vi "Controller Request PS Setpoints.vi"(8 "error in":errorcluster, 11 "Return All Setpoints":bool) -> (0 "error out":errorcluster)   [LabVIEW 2011, in "Controller VIs.lvlib"]
uses:
  Controller VIs.lvlib
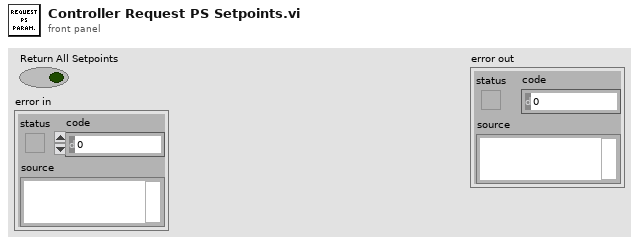
[diagram p1: front panel]
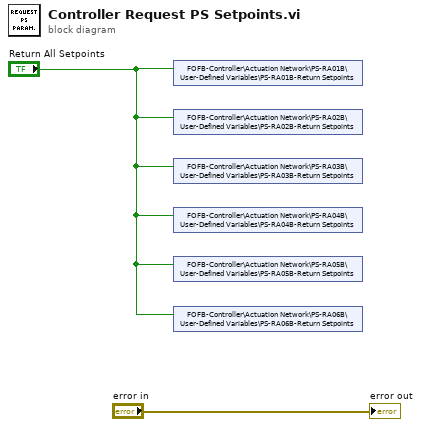
[diagram p0: block diagram]
diagram:
  n1 = shared-variable "FOFB-Controller\\Actuation Network\\PS-RA01B\\User-Defined Variables\\PS-RA01B-Return Setpoints"("Return All Setpoints") -> ()  [unwired: 1 in, 1 out]
  n2 = shared-variable "FOFB-Controller\\Actuation Network\\PS-RA02B\\User-Defined Variables\\PS-RA02B-Return Setpoints"("Return All Setpoints") -> ()  [unwired: 1 in, 1 out]
  n3 = shared-variable "FOFB-Controller\\Actuation Network\\PS-RA03B\\User-Defined Variables\\PS-RA03B-Return Setpoints"("Return All Setpoints") -> ()  [unwired: 1 in, 1 out]
  n4 = shared-variable "FOFB-Controller\\Actuation Network\\PS-RA04B\\User-Defined Variables\\PS-RA04B-Return Setpoints"("Return All Setpoints") -> ()  [unwired: 1 in, 1 out]
  n5 = shared-variable "FOFB-Controller\\Actuation Network\\PS-RA05B\\User-Defined Variables\\PS-RA05B-Return Setpoints"("Return All Setpoints") -> ()  [unwired: 1 in, 1 out]
  n6 = shared-variable "FOFB-Controller\\Actuation Network\\PS-RA06B\\User-Defined Variables\\PS-RA06B-Return Setpoints"("Return All Setpoints") -> ()  [unwired: 1 in, 1 out]
  "error out" <- "error in"
